vi "Control Tenma supply voltage.vi"() -> ()   [LabVIEW 2022 SP3]
uses:
  ADAM Serial/Instrument drivers/TENMA 72-2xxx PSU/ctls/TENMA 72-2xxx commands.ctl
panel:
  out "Returned string":string
  out "Returned value":sgl=nan format="%_4g"
  out "Output enabled":bool
  out "CV mode":bool
  out "Error out":errorcluster
  in  "Voltate output (V)":sgl=24.0
  in  "Port":refnum<visa-resource-name>="COM18"
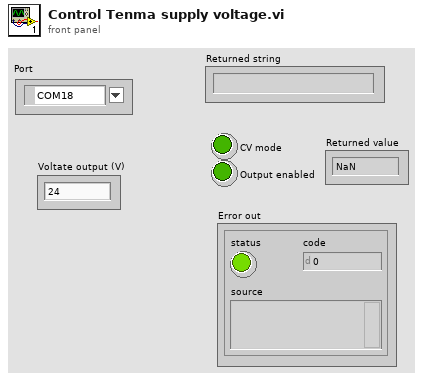
[diagram p1: front panel]
types:
  T1 = typedef "TENMA 72-2xxx commands.ctl" = string
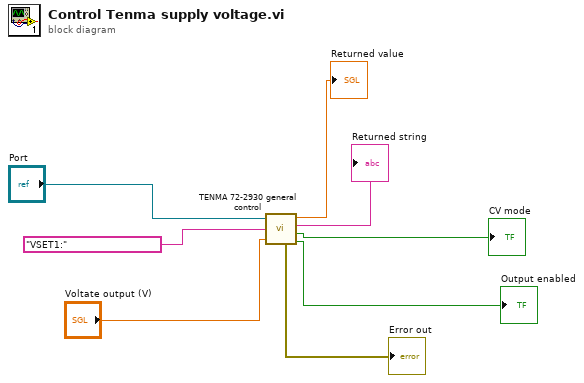
[diagram p0: block diagram]
diagram:
  n1 = call "TENMA 72-2930 general control.vi"("Value to set"="Voltate output (V)", "Command"=T1 "VSET1:", "Port"="Port") -> ("Output enabled"=→"Output enabled":bool, "error out"=→"Error out":errorcluster, "CV mode"=→"CV mode":bool, "Returned string"=→"Returned string":string, "Returned value"=→"Returned value":sgl)  [unwired: 1 in]
